vi "Panther Dashboard for DQMH.vi"(8 "error in":errorcluster) -> (0 "error out":errorcluster)   [LabVIEW 2021]
doc: "Start Panther Dashboard for DQMH\n\nScan the project caller for DQMH Modules\nShow the front panel"
uses:
  Panther Dashboard/Panther Dashboard/Panther Dashboard.lvlib
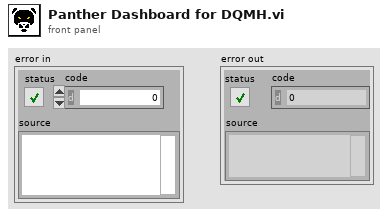
[diagram p1: front panel]
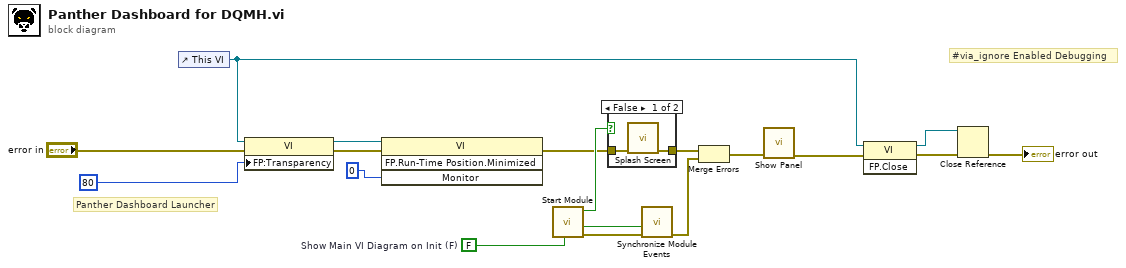
[diagram p0: block diagram]
diagram:
  w13 = FALSE  # Show Main VI Diagram on Init (F)
  # "#via_ignore Enabled Debugging"
  # "Panther Dashboard Launcher"
  n1 = control-ref of="This VI"() -> (w9:refnum<vi>)
  n2 = property class="VI"(reference=w9, error in="error in", "FP:Transparency"=u8 80 ("Front Panel Window:Transparency")) -> (reference out=w10:refnum<vi>, error out=w17:errorcluster)
  n3 = invoke class="VI" method="FP.Run-Time Position.Minimized"(reference=w10, error in=w17, "Monitor"=i16 0) -> (error out=w6:errorcluster)  [unwired: 1 in, 3 out]
  n4 = call "Start Module.vi"("Show Main VI Diagram on Init (F)"=w13) -> ("error out"=w5:errorcluster, "Wait for Event Sync?"=w14:bool, "Module Was Already Running?"=w7:bool)  [unwired: 7 in, 1 out]
  n5 = case shown="False" w7 {
    tunnel: w6 -> [w20 w21]
    tunnel: [w19 w21] -> w4
    frame False {
      n6 = call "Splash Screen.vi"("error in"=w20) -> ("error out"=w19:errorcluster)  [unwired: 10 in]
    }
    frame True {
    }
  }
  n7 = call "Synchronize Module Events.vi"("error in"=w5, "Wait for Event Sync?"=w14) -> ("error out"=w16:errorcluster)  [unwired: 9 in]
  n8 = Merge Errors(w4, w16) -> (w2:errorcluster)
  n9 = call "Show Panel.vi"("error in (no error)"=w2) -> ("error out"=w1:errorcluster)  [unwired: 10 in]
  n10 = invoke class="VI" method="FP.Close"(reference=w9, error in=w1) -> (reference out=w8:refnum<vi>, error out=w18:errorcluster)  [unwired: 1 in, 1 out]
  n11 = Close Reference(reference=w8, error in (no error)=w18) -> (error out=→"error out":errorcluster)
